vi "DCMotorResetFailsafe.vi"(0 "error in (no error)":errorcluster, 3 "Device In":u64) -> (7 "error out":errorcluster, 10 "Device Out":u64)   [LabVIEW 2012, in "Phidget DC Motor.lvlib"]
doc: "${ResetFailsafe:Header}"
uses:
  <instrlib>/Phidgets/Phidget DC Motor/Phidget DC Motor.lvlib
  <instrlib>/Phidgets/Phidget Common/Phidget Common.lvlib
  phidget22.dll
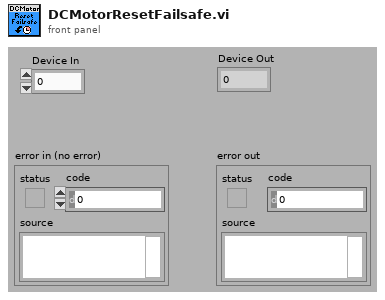
[diagram p1: front panel]
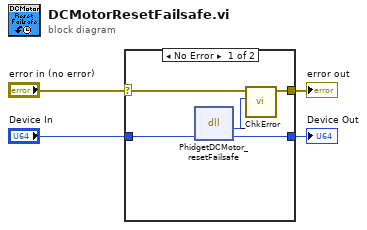
[diagram p0: block diagram]
diagram:
  n1 = case shown="No Error" "error in (no error)" {
    selector: "error in (no error)" -> [w7 w11]
    tunnel: [w6 w11] -> w3
    tunnel: "Device In" -> [w9 w10]
    tunnel: [w8 w10] -> w1
    frame No Error {
      n2 = dll-call lib="phidget22.*" fn="PhidgetDCMotor_resetFailsafe"("phid"=w9) -> ("return type"=w5:i32, "phid"=w8:u64)  [unwired: 3 in, 2 out]
      n3 = call <instrlib>:"_ChkError.vi"("Return Code"=w5, "error in (no error)"=w7) -> ("error out"=w6:errorcluster)  [unwired: 9 in]
    }
    frame Error {
    }
  }
  "error out" <- w3
  "Device Out" <- w1
